vi "PacLims.vi"(0 "param (in)":T1={"Srated"=25000.0, "eta [pu]"=0.98, "model"={"in-states"={"v1"=0.0, "v2"=0.0, "SoC"=0.0}, "output"={"V"=0.0, "Zeq"=0.0, "Eeq"=0.0}}} {"model"."output"."Eeq" format="%#.6g"; "model"."output"."Zeq" format="%#.6g"; "eta [pu]" format="%#_13g"}) -> (1 "PacLims":cluster{"Pmax":dbl, "Pmin":dbl} {"Pmax" format="%#.6g"; "Pmin" format="%#.6g"}, 2 "param (out)":T1={"Srated"=25000.0, "eta [pu]"=0.98, "model"={"in-states"={"v1"=0.0, "v2"=0.0, "SoC"=0.0}, "output"={"V"=0.0, "Zeq"=0.0, "Eeq"=0.0}}} {"model"."output"."Eeq" format="%#.6g"; "model"."output"."Zeq" format="%#.6g"; "eta [pu]" format="%#_13g"}, 3 "Ilims":cluster{"i(Pmax)":dbl, "i(Pmin)":dbl})   [LabVIEW 2021]
uses:
  General purpose/agent-variables.ctl
panel:
  in  "dc lims":T2={"vmax"=610.0, " vmin"=481.0, "imax"=41.0, "imin"=-41.0}
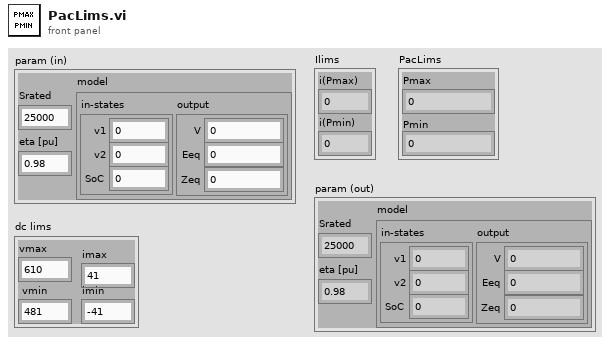
[diagram p1: front panel]
types:
  T1 = typedef "agent-variables.ctl" = cluster{"Srated":dbl, "eta [pu]":dbl, "model":cluster{"in-states":cluster{"v1":dbl, "v2":dbl, "SoC":dbl}, "output":cluster{"V":dbl, "Zeq":dbl, "Eeq":dbl}}}
  T2 = cluster{"vmax":dbl, " vmin":dbl, "imax":dbl, "imin":dbl}
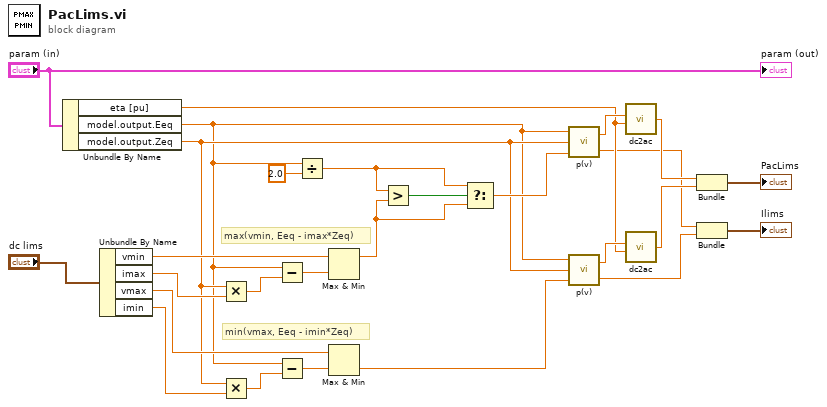
[diagram p0: block diagram]
diagram:
  # "max(vmin, Eeq - imax*Zeq)"
  # "min(vmax, Eeq - imin*Zeq)"
  n1 = Unbundle By Name("param (in)") -> ("eta [pu]"=w8:dbl, "model.output.Eeq"=w5:dbl, "model.output.Zeq"=w6:dbl)
  n2 = Unbundle By Name("dc lims") -> ("vmin"=w11:dbl, "imax"=w10:dbl, "vmax"=w9:dbl, "imin"=w7:dbl)
  n3 = Multiply(x=w6, y=w10) -> (x*y=w25:dbl)
  n4 = Multiply(x=w6, y=w7) -> (x*y=w23:dbl)
  n5 = Subtract(x=w5, y=w25) -> (x-y=w24:dbl)
  n6 = Subtract(x=w5, y=w23) -> (x-y=w22:dbl)
  n7 = Divide(x=w5, y=2.0) -> (x/y=w19:dbl)
  n8 = Max & Min(x=w11, y=w24) -> (max(x,y)=w16:dbl)  [unwired: 1 out]
  n9 = Max & Min(x=w9, y=w22) -> (min(x,y)=w17:dbl)  [unwired: 1 out]
  n10 = Greater?(x=w19, y=w16) -> (0:w20:bool)
  n11 = Select(t=w19, s=w20, f=w16) -> (s? t:f=w18:dbl)
  n12 = call "p(v).vi"("v"=w18, "Z"=w6, "E"=w5) -> ("i"=w3:dbl, "p"=w15:dbl)
  n13 = call "p(v).vi"("v"=w17, "Z"=w6, "E"=w5) -> ("i"=w4:dbl, "p"=w14:dbl)
  n14 = call "dc2ac.vi"("Efficiency [pu]"=w8, "Pdc"=w15) -> ("Pac"=w13:dbl)  [unwired: 2 in]
  n15 = call "dc2ac.vi"("Efficiency [pu]"=w8, "Pdc"=w14) -> ("Pac"=w27:dbl)  [unwired: 2 in]
  n16 = Bundle("Pac"=w13, "Pac"=w27) -> (→"PacLims":cluster{"Pac":dbl, "Pac":dbl})  [unwired: 1 in]
  n17 = Bundle("i"=w3, "i"=w4) -> (→"Ilims":cluster{"i":dbl, "i":dbl})  [unwired: 1 in]
  "param (out)" <- "param (in)"
